vi "testUtility.vi"(8 "error in (no error)":errorcluster) -> (0 "error out":errorcluster)   [LabVIEW 2018]
doc: "Test all test cases from Utility directory."
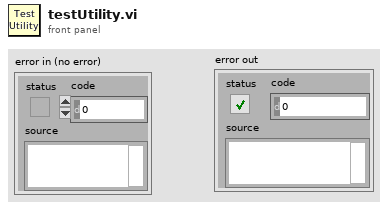
[diagram p1: front panel]
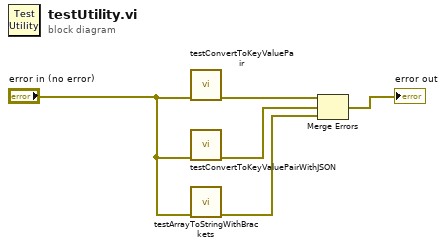
[diagram p0: block diagram]
diagram:
  n1 = call "testConvertToKeyValuePair.vi"("error in (no error)"="error in (no error)") -> ("error out"=w5:errorcluster)  [unwired: 10 in]
  n2 = call "testConvertToKeyValuePairWithJSON.vi"("error in (no error)"="error in (no error)") -> ("error out"=w4:errorcluster)  [unwired: 10 in]
  n3 = call "testArrayToStringWithBrackets.vi"("error in (no error)"="error in (no error)") -> ("error out"=w2:errorcluster)  [unwired: 10 in]
  n4 = Merge Errors(w5, w4, w2) -> (→"error out":errorcluster)
